vi "Save_coutoutALL.vi"(0 "configuration file path":path caption="配置文件的路径", 1 "测试信息 2":refnum<vi>, 5 "error in (no error)":errorcluster caption="错误输入（无错误）") -> (14 "添加的路径":path, 19 "error out":errorcluster caption="错误输出")   [LabVIEW 2018]
uses:
  <vilib>/Utility/config.llb/Write Key (String).vi
  <vilib>/Utility/config.llb/NI_LVConfig.lvlib
panel:
  out "key names":string[](array[string]) caption="键名"
  out "子数组":string[](array[string])
  in  "测试信息":i32(listbox)
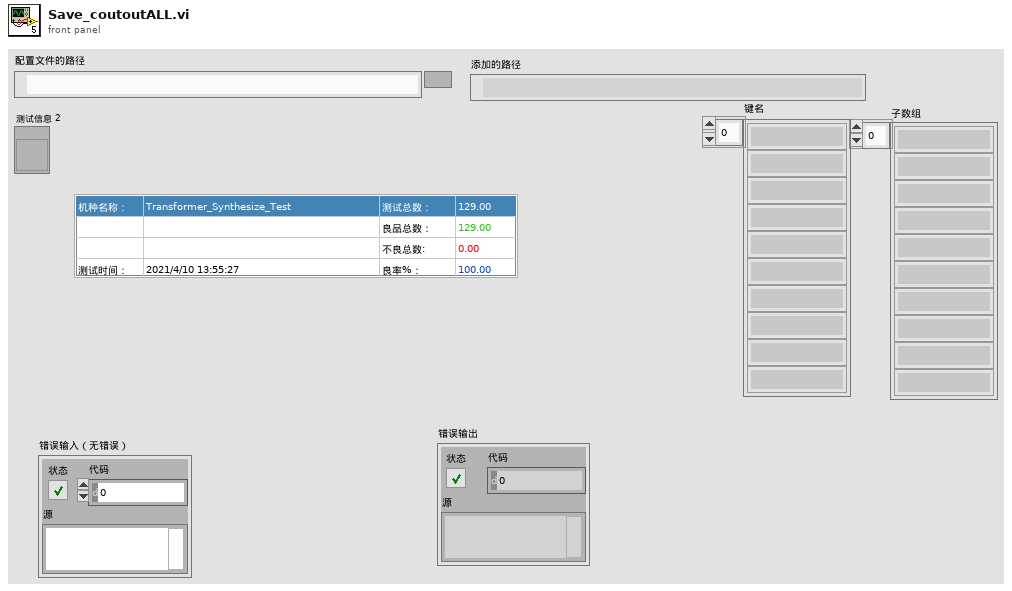
[diagram p1: front panel]
types:
  T1 = typedef "NI_LVConfig.lvlib/Config Data RefNum.ctl" = refnum<k1>
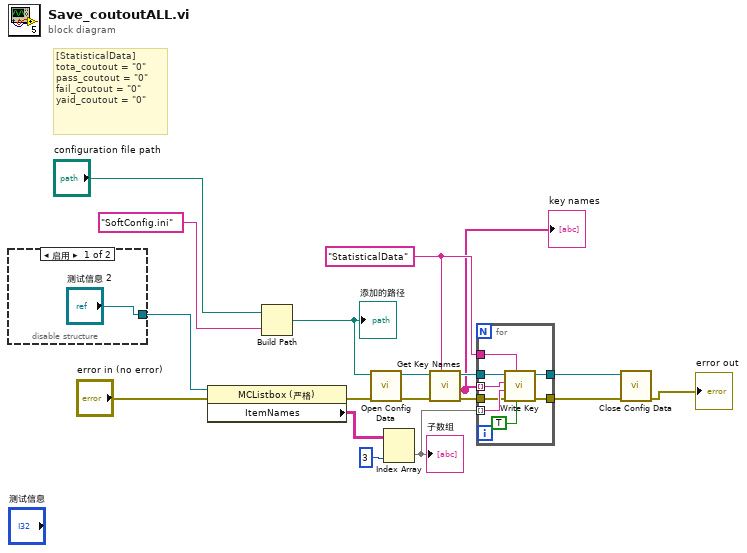
[diagram p0: block diagram]
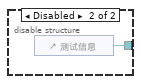
[diagram p2: hidden frame]
diagram:
  w14 = "StatisticalData" ("section")
  # "[StatisticalData]\ntota_coutout = \"0\"\npass_coutout = \"0\"\nfail_coutout = \"0\"\nyaid_coutout = \"0\""
  n1 = disable-structure shown="启用" {
    disable-tunnel: ["测试信息 2" w20] -> w11
    frame Enabled {
    }
    frame Disabled {
      n2 = control-ref of="测试信息"() -> (w20:refnum<vi>)
    }
  }
  n3 = property class="MCListbox (严格)"(reference=w11, error in="error in (no error)") -> (error out=w6:errorcluster, "ItemNames"=w10:string[][])  [unwired: 1 out]
  n4 = Build Path(base path="configuration file path", name or relative path="SoftConfig.ini" ("名称或相对路径")) -> (appended path=w18:path)
  "添加的路径" <- w18
  n5 = call <vilib>:"Open Config Data.vi"("error in (no error)"=w6, "configuration file path"=w18) -> ("error out"=w7:errorcluster, "refnum"=w12:T1)  [unwired: 7 in, 1 out]
  n6 = Index Array(array=w10, index (col)=3 ("禁用的索引 (列)")) -> (element=w8:string[])  [unwired: 1 in]
  "子数组" <- w8
  n7 = call <vilib>:"Get Key Names.vi"("section"=w14, "error in (no error)"=w7, "refnum"=w12) -> ("error out"=w5:errorcluster, "key names"=w13:string[], "refnum out"=w15:T1)  [unwired: 5 in, 1 out]
  "key names" <- w13
  n8 = for {
    tunnel: w13 -> [w27] mode=indexing
    tunnel: w14 -> [w28]
    tunnel: w15 -> [w26]
    tunnel: w8 -> [w25] mode=indexing
    tunnel: w5 -> [w24]
    tunnel: [w23] -> w2
    tunnel: [w21] -> w3
    n9 = call-poly <vilib>:"Write Key.vi"("write raw string? (F)"=TRUE, "section"=w28, "error in (no error)"=w24, "value"=w25, "key"=w27, "refnum"=w26) -> ("error out"=w23:errorcluster, "refnum out"=w21:T1)  [unwired: 3 in, 1 out]
  }
  n10 = call <vilib>:"Close Config Data.vi"("error in (no error)"=w2, "refnum"=w3) -> ("error out"=→"error out":errorcluster)  [unwired: 8 in, 1 out]
